vi "Set Thermocouple Type.vi"(8 "error in (no error)":errorcluster, 10 "Thermocouple Type":T1, 11 "Grove Thermocouple MCP9600 in":refnum<class "Grove Thermocouple MCP9600.lvclass">) -> (0 "error out":errorcluster, 3 "Grove Thermocouple MCP9600 out":refnum<class "Grove Thermocouple MCP9600.lvclass">)   [LabVIEW 2020, in "CTI-Peripheral.lvlib" / "Grove Thermocouple MCP9600.lvclass"]
uses:
  Grove Thermocouple MCP9600.lvclass
  Controls/ThermocoupleType.ctl
  Grove Thermocouple MCP9600.lvclass/Grove Thermocouple MCP9600.ctl
  CTI/I2C Connection/I2C Connection.lvclass/I2C Connection.ctl
  CTI/Session/I2C Write Data.vi
  CTI/I2C Connection/I2C Connection.lvclass
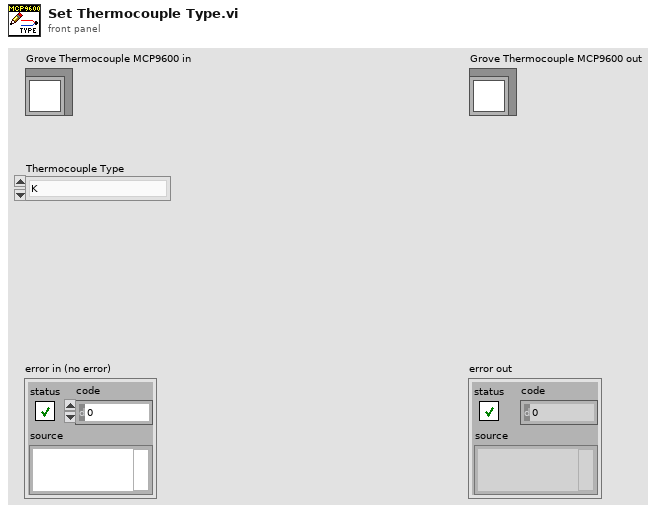
[diagram p1: front panel]
types:
  T1 = typedef "CTI-Peripheral.lvlib/Grove Thermocouple MCP9600.lvclass/ThermocoupleType.ctl" = enum16{"K", "J", "T", "N", "S", "E", "B", "R"}
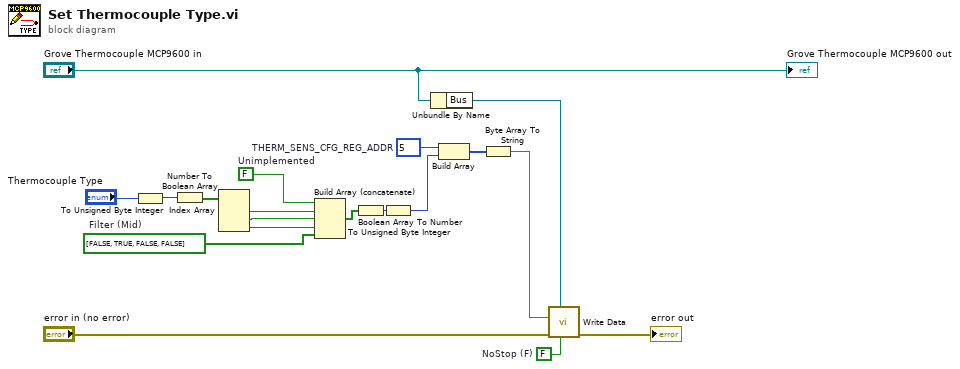
[diagram p0: block diagram]
diagram:
  w6 = FALSE  # NoStop (F)
  w8 = bool[] [FALSE, TRUE, FALSE, FALSE]  # Filter (Mid)
  w12 = FALSE  # Unimplemented
  w19 = u8 5  # THERM_SENS_CFG_REG_ADDR
  n1 = To Unsigned Byte Integer(number="Thermocouple Type") -> (unsigned 8bit integer=w17:u8)
  n2 = Number To Boolean Array(number=w17) -> (Boolean array=w16:bool[])
  n3 = Index Array(array=w16) -> (element #1=w15:bool, element #2=w14:bool, element #3=w13:bool)  [unwired: 3 in]
  n4 = Build Array (concatenate)(w12, w15, w14, w13, w8) -> (w11:bool[])
  n5 = Boolean Array To Number(Boolean array=w11) -> (number=w10:u32)
  n6 = To Unsigned Byte Integer(number=w10) -> (unsigned 8bit integer=w9:u8)
  n7 = Unbundle By Name("Grove Thermocouple MCP9600 in") -> ("Bus"=w1:refnum<class "I2C Connection.lvclass">)
  n8 = Build Array(w19, w9) -> (w18:u8[])
  n9 = Byte Array To String(unsigned byte array=w18) -> (string=w3:string)
  n10 = call "Write Data.vi"("NoStop (F)"=w6, "I2C Connection"=w1, "error in (no error)"="error in (no error)", "Data"=w3) -> ("error out"=→"error out":errorcluster)  [unwired: 7 in]
  "Grove Thermocouple MCP9600 out" <- "Grove Thermocouple MCP9600 in"
